vi "Board Parameters List.vi"(8 "error in (no error)":errorcluster, 11 "BoardHandle":T1) -> (0 "error out":errorcluster, 1 "Alarm bits":string[](array[string]), 2 "Parameters list":string[](array[string]), 3 "BoardHandle out":T1)   [LabVIEW 2020, in "CAEN PSM.lvlib"]
doc: "This function returns the list of board parameters supported by the device."
uses:
  CAEN PSM.lvlib
  Private/BoardHandle.ctl
  Private/DeviceFamily.ctl
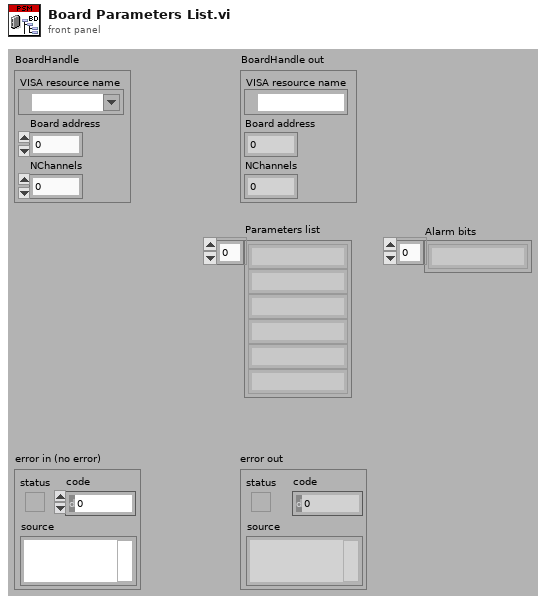
[diagram p1: front panel]
types:
  T1 = typedef "CAEN PSM.lvlib/BoardHandle.ctl" = cluster{"VISA resource name":refnum<visa-resource-name>, "Board address":i8, "NChannels":u8}
  T2 = typedef "CAEN PSM.lvlib/DeviceFamily.ctl" = enum8{"NIM / DESKTOP HV", "DT55XXE HV", "SMART HV"}
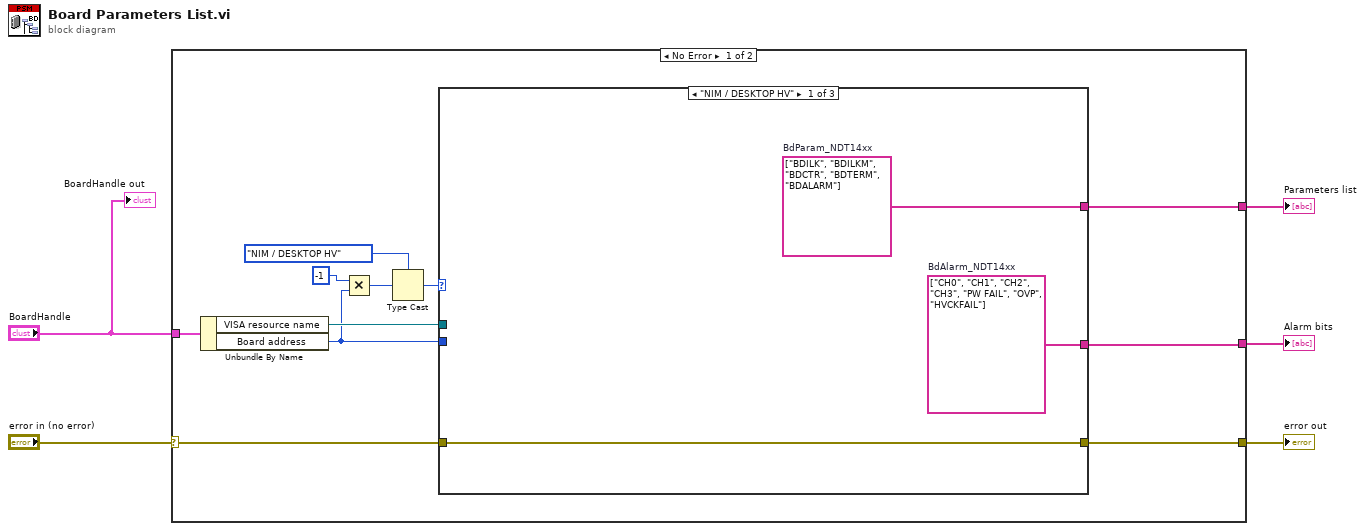
[diagram p0: block diagram]
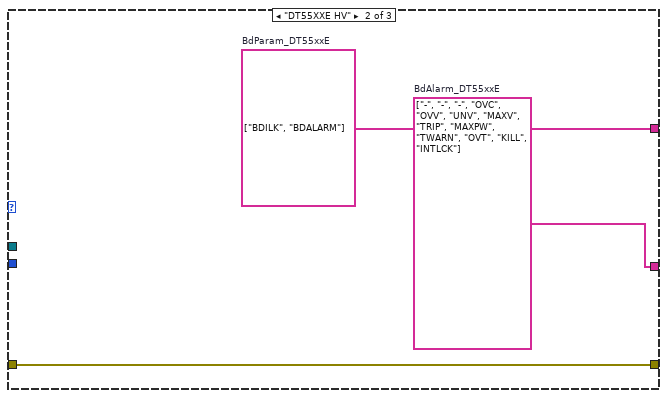
[diagram p2: hidden frame]
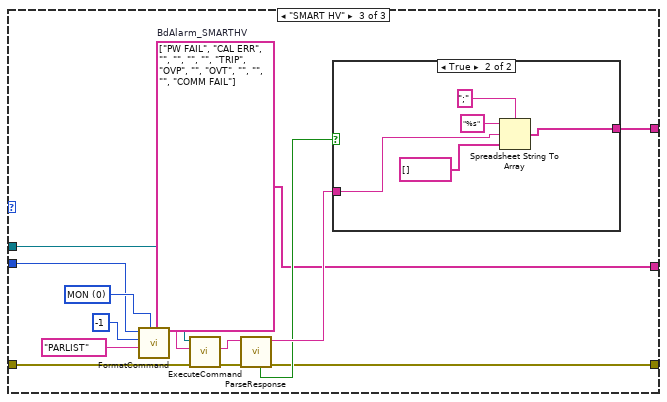
[diagram p3: hidden frame]
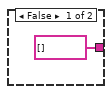
[diagram p4: hidden frame]
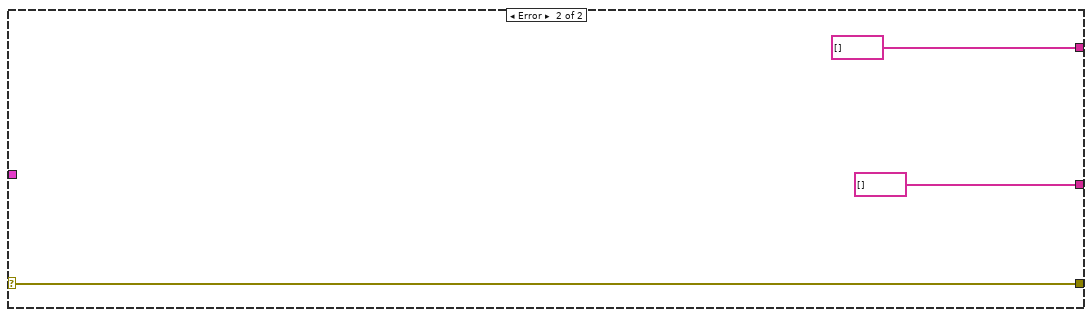
[diagram p5: hidden frame]
diagram:
  n1 = case shown="No Error" "error in (no error)" {
    selector: "error in (no error)" -> [w15 w45]
    tunnel: [w12 w45] -> w4
    tunnel: "BoardHandle" -> [w16 _]
    tunnel: [w13 string[] [] ("Parameters list")] -> w2
    tunnel: [w8 string[] [] ("BdStatus_SMARTHV")] -> w1
    frame No Error {
      n2 = Unbundle By Name(w16) -> ("VISA resource name"=w14:refnum<visa-resource-name>, "Board address"=w10:i8)
      n3 = Multiply(x=i8 -1, y=w10) -> (x*y=w7:i8)
      n4 = Type Cast(type=DeviceFamily."NIM / DESKTOP HV" ("Device Family"), x=w7) -> (*(type *) &x=w11:T2)
      n5 = case shown="\"NIM / DESKTOP HV\"" w11 {
        tunnel: w15 -> [w19 w21 w32]
        tunnel: w14 -> [_ _ w30]
        tunnel: w10 -> [_ _ w29]
        tunnel: [w18 w22 w26] -> w13
        tunnel: [w19 w21 w24] -> w12
        tunnel: [w17 w20 w23] -> w8
        frame "NIM / DESKTOP HV" {
          w17 = string[] ["CH0", "CH1", "CH2", "CH3", "PW FAIL", "OVP", "HVCKFAIL"]  # BdAlarm_NDT14xx
          w18 = string[] ["BDILK", "BDILKM", "BDCTR", "BDTERM", "BDALARM"]  # BdParam_NDT14xx
        }
        frame "DT55XXE HV" {
          w20 = string[] ["-", "-", "-", "OVC", "OVV", "UNV", "MAXV", "TRIP", "MAXPW", "TWARN", "OVT", "KILL", "INTLCK"]  # BdAlarm_DT55xxE
          w22 = string[] ["BDILK", "BDALARM"]  # BdParam_DT55xxE
        }
        frame "SMART HV" {
          w23 = string[] ["PW FAIL", "CAL ERR", "", "", "", "", "TRIP", "OVP", "", "OVT", "", "", "", "COMM FAIL"]  # BdAlarm_SMARTHV
          w36 = u8 0 items=["MON", "SET"] ("CMD")
          n6 = call "FormatCommand.vi"("CMD (MON)"=w36, "PAR"="PARLIST", "CH"=i8 -1, "BD (0)"=w29) -> ("cmd"=w35:string)  [unwired: 7 in]
          n7 = call "ExecuteCommand.vi"("error in (no error)"=w32, "Command"=w35, "VISA resource name"=w30) -> ("error out"=w34:errorcluster, "Response"=w33:string)  [unwired: 6 in, 1 out]
          n8 = call "ParseResponse.vi"("error in (no error)"=w34, "Response"=w33) -> ("error out"=w24:errorcluster, "val"=w27:string, "OK"=w25:bool)  [unwired: 6 in, 1 out]
          n9 = case shown="True" w25 {
            tunnel: w27 -> [_ w40]
            tunnel: [string[] [] ("array type (2D Dbl)") w38] -> w26
            frame False {
            }
            frame True {
              n10 = Spreadsheet String To Array(delimiter (Tab)=";", format string="%s", spreadsheet string=w40, array type (2D Dbl)=string[] []) -> (array=w38:string[])
            }
          }
        }
      }
    }
    frame Error {
    }
  }
  "error out" <- w4
  "Parameters list" <- w2
  "Alarm bits" <- w1
  "BoardHandle out" <- "BoardHandle"
